vi "dummy sender.vi"() -> ()   [LabVIEW 2021]
panel:
  in  "Boolean":bool
  in  "loop 1":i32
  out "Numeric 3":dbl
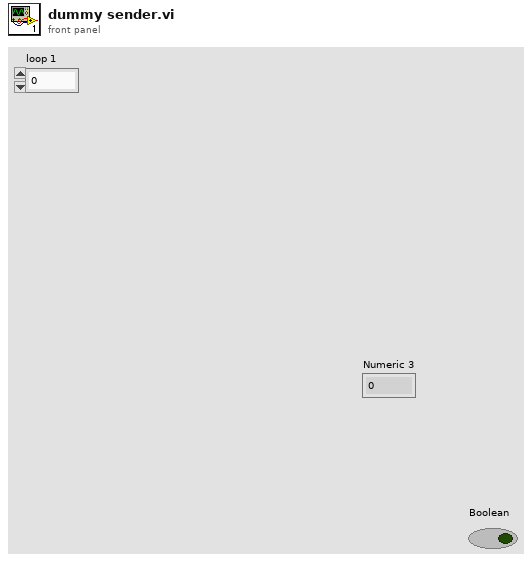
[diagram p1: front panel]
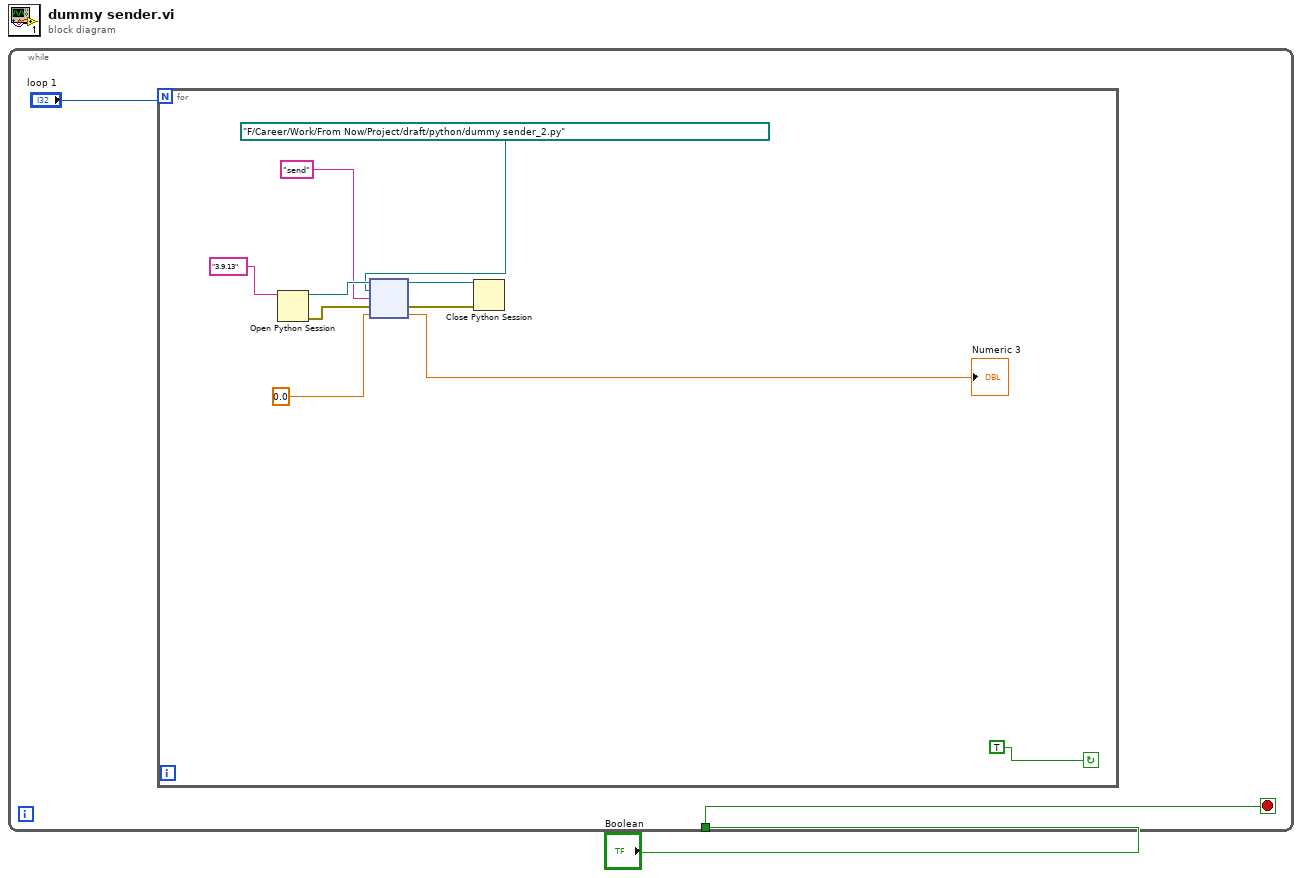
[diagram p0: block diagram]
diagram:
  n1 = while {
    tunnel: "Boolean" -> [w3]
    stop <- w3 stop-if-true
    n2 = for {
      N: "loop 1" -> [_]
      stop <- TRUE continue-if-true
      n3 = Open Python Session(python version="3.9.13" ("Python version")) -> (session out=w9:refnum<k35>, error out=w12:errorcluster)  [unwired: 2 in]
      n4 = node(w9, path "F:/Career/Work/From Now/Project/draft/python/dummy sender_2.py" ("module path"), "send" ("function name"), w12, 0.0) -> (w10:refnum<k35>, w11:errorcluster, →"Numeric 3":dbl)  [unwired: 2 out]
      n5 = Close Python Session(session in=w10, error in=w11) -> ()  [unwired: 1 out]
    }
  }
